vi "Open.vi"(7 "I2C Channel (0)":u8, 8 "Error In":errorcluster, 10 "ADXL345 Address":T1, 11 "LINX Resource":T2) -> (0 "Error Out":errorcluster, 3 "LINX Resource":T2)   [LabVIEW 2011, in "LVH-LINX.lvlib" / "ADXL345.lvlib"]
doc: "Initialize the ADXL345 and bring it out of sleep mode."
uses:
  ADXL345.lvlib
  Private/Type Defs/LINX Ref.ctl
  Private/Type Defs/Platform.ctl
  Private/Type Defs/Interface.ctl
  Private/Device/Type Defs/LINX Device Config.ctl
  Private/Device/Type Defs/TCP Config.ctl
  Private/Type Defs/Device Family.ctl
  Private/Device/Type Defs/Channels.ctl
  Address.ctl
  LVH-LINX.lvlib
  Private/Device/Device.lvlib
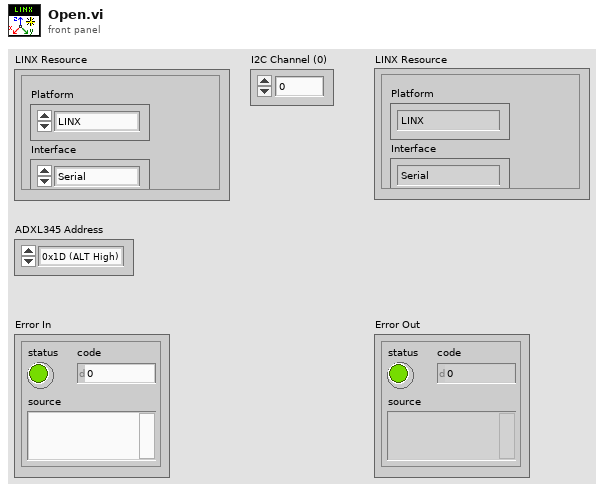
[diagram p1: front panel]
types:
  T1 = typedef "LVH-LINX.lvlib/ADXL345.lvlib/Address.ctl" = enum16{"0x1D (ALT High)", "0x53 (ALT Low)"}
  T2 = typedef "LVH-LINX.lvlib/LINX Ref.ctl" = cluster{"Platform":T3, "Interface":T4, "LINX Device Config":T5}
  T3 = typedef "LVH-LINX.lvlib/Platform.ctl" = enum16{"LINX", "myRIO"}
  T4 = typedef "LVH-LINX.lvlib/Interface.ctl" = enum16{"Serial", "TCP"}
  T5 = typedef "LVH-LINX.lvlib/Device.lvlib/LINX Device Config.ctl" = cluster{"Interface":T4, "COM Port":refnum<visa-resource-name>, "TCP Configuration":T6, "Device Family":T7, "Device ID":u8, "Device Name":string, "TCP Ref":refnum<k5>, "Channels":T8}
  T6 = typedef "LVH-LINX.lvlib/Device.lvlib/TCP Config.ctl" = cluster{"IP Address":string, "Port":u16}
  T7 = typedef "LVH-LINX.lvlib/Device Family.ctl" = enum8{"National Instruments", "Digilent", "Arduino"}
  T8 = typedef "LVH-LINX.lvlib/Channels.ctl" = cluster{"DI Channels":u8[], "DO Channels":u8[], "AI":u8[], "AO":u8[], "PWM":u8[], "QE":u8[], "UART":u8[], "I2C 2":u8[], "SPI":u8[], "CAN":u8[], "AI Ref (V)":dbl, "AO Resolution (Bits)":u8, "AO Ref (V)":dbl}
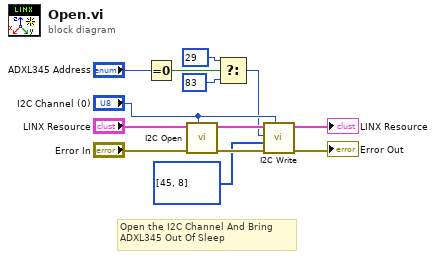
[diagram p0: block diagram]
diagram:
  # "Open the I2C Channel And Bring \nADXL345 Out Of Sleep"
  n1 = Equal To 0?(x="ADXL345 Address") -> (x = 0?=w6:bool)
  n2 = call "I2C Open.vi"("I2C Channel (0)"="I2C Channel (0)", "Error In"="Error In", "LINX Resource"="LINX Resource") -> ("Error Out"=w12:errorcluster, "LINX Resource"=w13:T2)  [unwired: 7 in]
  n3 = Select(t=u8 29 ("I2C Slave Address (0)"), s=w6, f=u8 83 ("I2C Slave Address (0)")) -> (s? t:f=w2:u8)
  n4 = call "I2C Write.vi"("I2C Channel"="I2C Channel (0)", "Error In"=w12, "Data"=u8[] [45, 8], "I2C Slave Address (0)"=w2, "LINX Resource"=w13) -> ("Error Out"=→"Error Out":errorcluster, "LINX Resource"=→"LINX Resource":T2)  [unwired: 5 in]
